vi "VIToEnv.vi"(0 "LabVIEW":refnum<vi>, 1 "Env In":variant, 2 "VI Path":path, 3 "Name":string, 4 "Options":i32=16 format="%.0x") -> (5 "Env Out":variant, 6 "VI Variant":variant)   [LabVIEW 2014]
uses:
  Env.global.vi
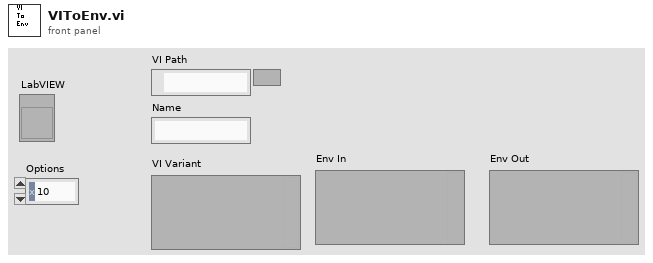
[diagram p1: front panel]
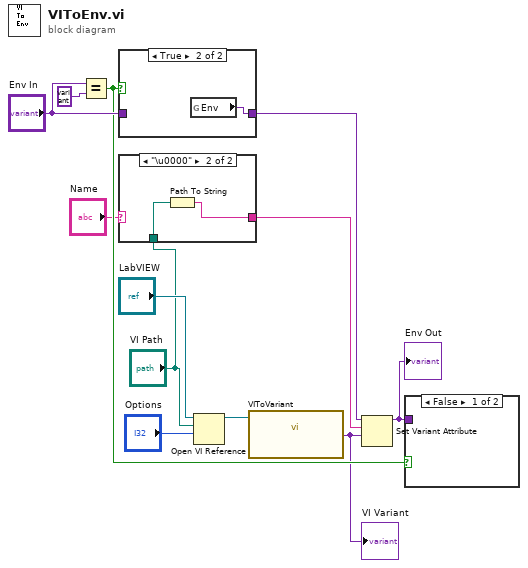
[diagram p0: block diagram]
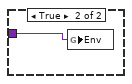
[diagram p3: hidden frame]
diagram:
  n1 = Equal?(x="Env In", y=variant ("Env In")) -> (x = y?=w8:bool)
  n2 = case shown="True" w8 {
    tunnel: [w13 w14] -> w10
    tunnel: "Env In" -> [w13 _]
    frame False {
    }
    frame True {
      n3 = global read "Env.global.vi" "Env"() -> (w14:variant)
    }
  }
  n4 = case shown="\"\"" "Name" {
    selector: "Name" -> [w15 _]
    tunnel: [w15 w16] -> w2
    tunnel: "VI Path" -> [_ w17]
    frame Default {
    }
    frame "\u0000" {
      n5 = Path To String(path=w17) -> (string=w16:string)
    }
  }
  n6 = Open VI Reference(application reference (local)="LabVIEW", vi path="VI Path", options="Options") -> (vi reference=w12:refnum<vi>)  [unwired: 3 in, 1 out]
  n7 = call "VIToVariant.vi"("VI Reference"=w12) -> ("VI Variant"=w6:variant)  [unwired: 1 in]
  "VI Variant" <- w6
  n8 = Set Variant Attribute(Variant=w10, name=w2, value=w6) -> (Variant out=w7:variant)  [unwired: 1 in, 2 out]
  "Env Out" <- w7
  n9 = case shown="False" w8 {
    tunnel: w7 -> [_ w18]
    frame False {
    }
    frame True {
      n10 = global write "Env.global.vi" "Env"(w18) -> ()
    }
  }
